vi "StartDatabase.vi"(8 "error in (no error)":errorcluster, 10 "SQL query":string, 11 "测试类型":string) -> (0 "error out 2":errorcluster)   [LabVIEW 2014]
uses:
  <vilib>/addons/database/Connection.llb/DB Tools Open Connec (String).vi
  <vilib>/addons/database/Connection.llb/Conn Execute.vi
  <vilib>/addons/database/Recordset.llb/Rec Destroy - Connection.vi
  <vilib>/addons/database/NI_Database_API.lvlib
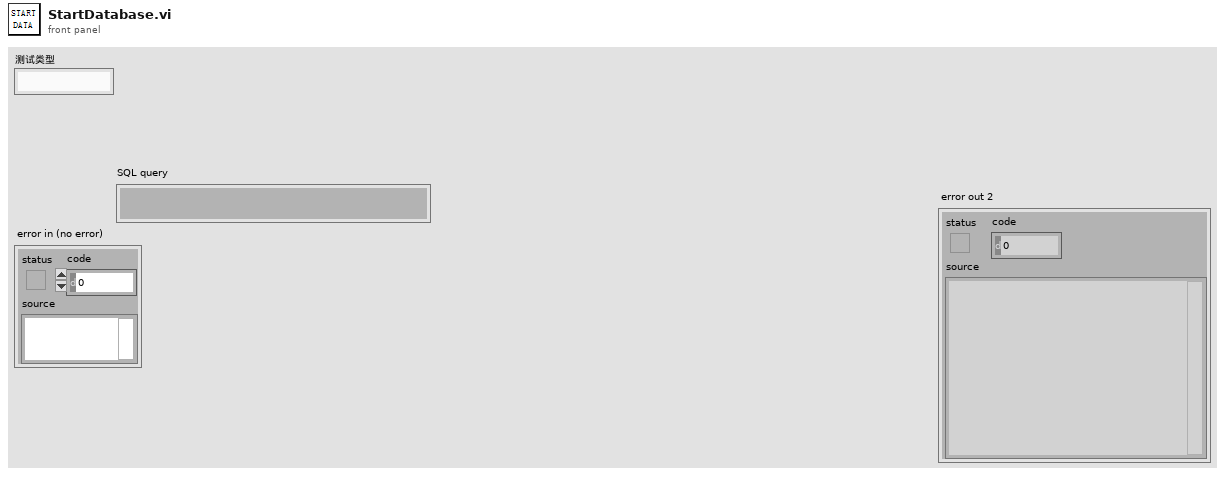
[diagram p1: front panel]
types:
  T1 = typedef "NI_Database_API.lvlib/Conn ObjectReference.ctl" = refnum<k1>
  T2 = typedef "NI_Database_API.lvlib/Rec ObjectReference.ctl" = refnum<k1>
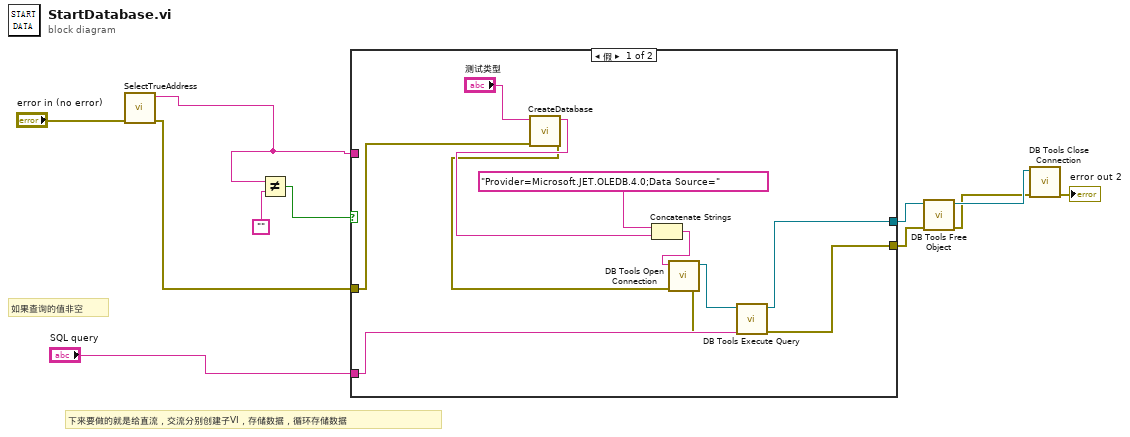
[diagram p0: block diagram]
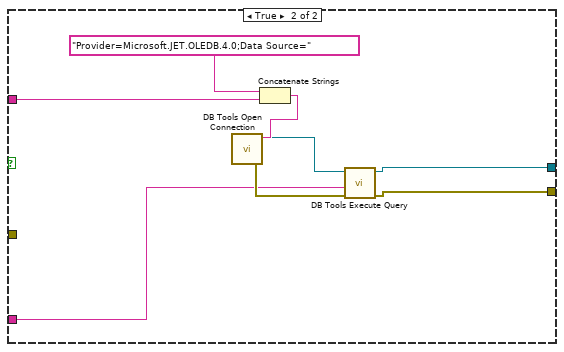
[diagram p2: hidden frame]
diagram:
  # "下来要做的就是给直流，交流分别创建子VI，存储数据，循环存储数据"
  # "如果查询的值非空"
  n1 = call "SelectTrueAddress.vi"("error in (no error)"="error in (no error)") -> ("error out"=w2:errorcluster, "元素"=w3:string)  [unwired: 9 in]
  n2 = Not Equal?(x=w3, y="") -> (x != y?=w4:bool)
  n3 = case shown="假" w4 {
    tunnel: "SQL query" -> [w19 w26]
    tunnel: [w14 w25] -> w7
    tunnel: [w13 w24] -> w6
    tunnel: w2 -> [w16 _]
    tunnel: w3 -> [_ w23]
    frame False {
      n4 = call "CreateDatabase.vi"("错误输入（无错误）"=w16, "测试类型"="测试类型") -> ("error out"=w15:errorcluster, "数据库地址"=w17:string)  [unwired: 8 in]
      n5 = Concatenate Strings("Provider=Microsoft.JET.OLEDB.4.0;Data Source=", w17) -> (w21:string)
      n6 = call-poly <vilib>:"DB Tools Open Connection.vi"("error in (no error)"=w15, "connection information"=w21) -> ("error out"=w18:errorcluster, "connection reference"=w20:T1)  [unwired: 6 in]
      n7 = call-poly <vilib>:"DB Tools Execute Query.vi"("error in (no error)"=w18, "SQL query"=w19, "connection reference"=w20) -> ("error out"=w13:errorcluster, "recordset reference"=w14:T2)  [unwired: 5 in]
    }
    frame True {
      n8 = Concatenate Strings("Provider=Microsoft.JET.OLEDB.4.0;Data Source=", w23) -> (w29:string)
      n9 = call-poly <vilib>:"DB Tools Open Connection.vi"("connection information"=w29) -> ("error out"=w27:errorcluster, "connection reference"=w28:T1)  [unwired: 7 in]
      n10 = call-poly <vilib>:"DB Tools Execute Query.vi"("error in (no error)"=w27, "SQL query"=w26, "connection reference"=w28) -> ("error out"=w24:errorcluster, "recordset reference"=w25:T2)  [unwired: 5 in]
    }
  }
  n11 = call-poly <vilib>:"DB Tools Free Object.vi"("error in (no error)"=w6, "recordset reference"=w7) -> ("error out"=w9:errorcluster, "connection reference"=w10:T1)  [unwired: 8 in]
  n12 = call <vilib>:"DB Tools Close Connection.vi"("error in (no error)"=w9, "connection reference"=w10) -> ("error out"=→"error out 2":errorcluster)  [unwired: 5 in]
